vi "Read Stop Notifier.vi"(8 "error in (no error)":errorcluster, 11 "Continue Running Task in":refnum<class "Continue Running Task.lvclass">) -> (0 "error out":errorcluster, 2 "Stop Notifier":T1, 3 "Continue Running Task out":refnum<class "Continue Running Task.lvclass">)   [LabVIEW 2019]
uses:
  Continue Running Task.lvclass
  C:/Users/iio/Desktop/NTHU Brain Center/General Library/Ancestor Class/Task/Task.lvclass
  Type Def/Stop Notifier.ctl
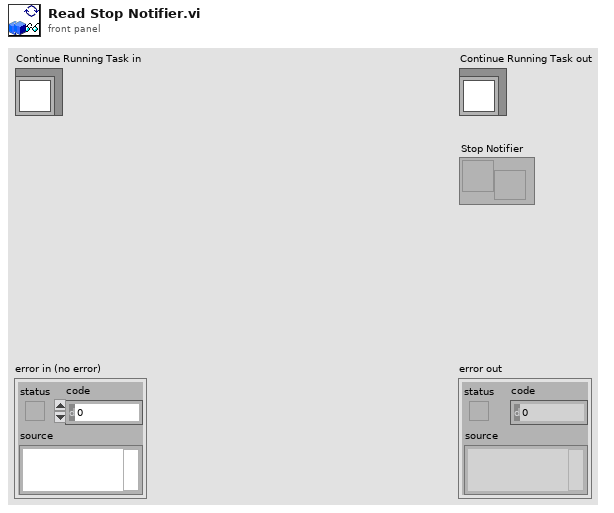
[diagram p1: front panel]
types:
  T1 = typedef "Stop Notifier.ctl" = refnum<notifier>
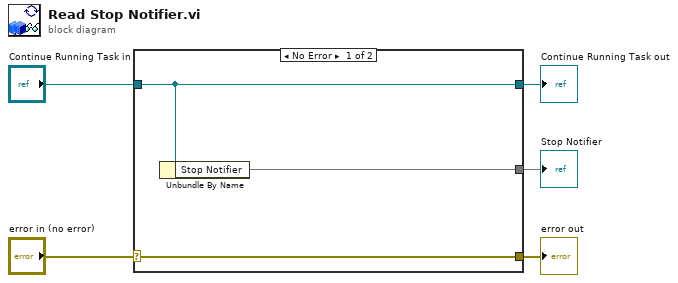
[diagram p0: block diagram]
diagram:
  n1 = case shown="No Error" "error in (no error)" {
    selector: "error in (no error)" -> [w8 w9]
    tunnel: [w8 w9] -> w4
    tunnel: [w7 w10] -> w2
    tunnel: "Continue Running Task in" -> [w7 w10]
    tunnel: [w6 _] -> w1
    frame No Error {
      n2 = Unbundle By Name(w7) -> ("Stop Notifier"=w6)
    }
    frame Error {
    }
  }
  "error out" <- w4
  "Continue Running Task out" <- w2
  "Stop Notifier" <- w1
